vi "报警信息记录.vi"(8 "error in (no error)":errorcluster, 10 "code":u64, 11 "Slave ID":T1=enum."氨氮") -> (0 "error out":errorcluster)   [LabVIEW 2016, in "质控单元V2.lvlib"]
uses:
  Alarm interface/Alarm interface.lvlib
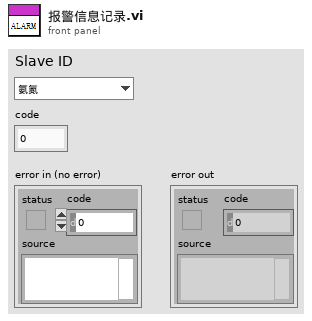
[diagram p1: front panel]
types:
  T1 = typedef "质控单元V2.lvlib/质控slave id.ctl" = enum16{"null", "氨氮", "总磷", "总氮", "CODMn", "CODCr"}
  T2 = typedef "Alarm interface.lvlib/map in.ctl" = cluster{"name":string, "CN":string, "FirmwareVersion":string, "code":string}
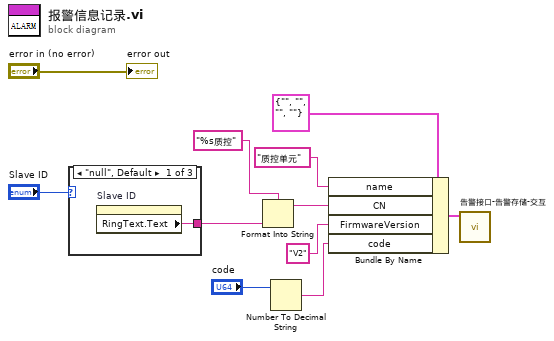
[diagram p0: block diagram]
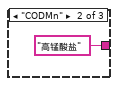
[diagram p2: hidden frame]
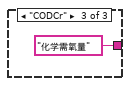
[diagram p3: hidden frame]
diagram:
  n1 = case shown="\"null\", Default" "Slave ID" {
    tunnel: [w12 "高锰酸盐" ("RingText.Text") "化学需氧量" ("RingText.Text")] -> w6
    frame "null", Default {
      n2 = property on="Slave ID" class="Enum (strict)"() -> ("RingText.Text"=w12:string)  [unwired: 2 in, 2 out]
    }
    frame "CODMn" {
    }
    frame "CODCr" {
    }
  }
  n3 = Format Into String(format string="%s质控" ("格式字符串"), w6) -> (resulting string=w4:string)  [unwired: 2 in, 1 out]
  n4 = Number To Decimal String(number="code") -> (decimal integer string=w2:string)  [unwired: 1 in]
  n5 = Bundle By Name(cluster=T2 {"name"="", "CN"="", "FirmwareVersion"="", "code"=""} ("map in"), "name"="质控单元", "CN"=w4, "FirmwareVersion"="V2", "code"=w2) -> (w3:T2)
  n6 = call "告警接口-告警存储-交互.vi"("map in"=w3) -> ()  [unwired: 10 in, 1 out]
  "error out" <- "error in (no error)"
